vi "Z to xyr.vi"(8 "Z":dbl=1.0 format="%#_13g", 11 "R":dbl=2.0 format="%#_13g") -> (1 "r":dbl, 2 "r/yc":dbl, 3 "xc":dbl)   [LabVIEW 2014]
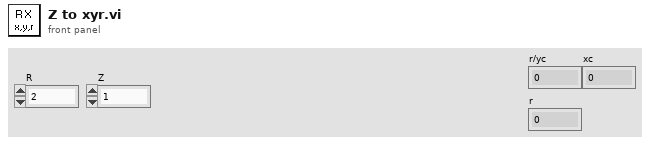
[diagram p1: front panel]
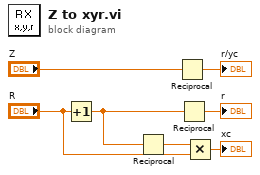
[diagram p0: block diagram]
diagram:
  n1 = Increment(x="R") -> (x+1=w4:dbl)
  n2 = Reciprocal(x=w4) -> (1/x=w3:dbl)
  n3 = Reciprocal(x="Z") -> (1/x=→"r/yc":dbl)
  n4 = Reciprocal(x=w4) -> (1/x=→"r":dbl)
  n5 = Multiply(x=w3, y="R") -> (x*y=→"xc":dbl)
